vi "Create.vi"(8 "Error In":errorcluster, 11 "object in":refnum<class "WebView.lvclass">) -> (0 "Error Out":errorcluster, 3 "object out":refnum<class "WebView.lvclass">)   [LabVIEW 2024, in "WebView.lvclass"]
uses:
  <resource>/Framework/Providers/Open_GDS/ClassProviders/Provider_LvNativeClass/Templates/NativeBaseTemplate_4x4x4/NativeBaseTemplate_4x4x4.lvclass/NativeBaseTemplate_4x4x4.ctl
  WebView.lvclass
  WebView.lvclass/WebView.ctl
  <vilib>/sklein/WebView2/Webview2 Control/Paths.ctl
  <vilib>/sklein/WebView2/Webview2 Control/WebView2 Control.xctl
  <vilib>/sklein/WebView2/Webview2 Control/Core Env Options.ctl
panel:
  in  "Environment Options":T1
  in  "Path Overrides":T2
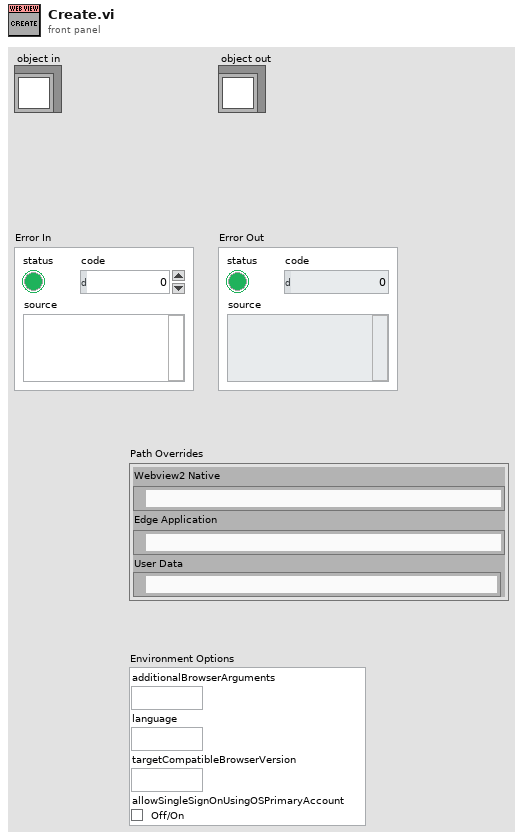
[diagram p1: front panel]
types:
  T1 = typedef "WebView2 Control.xctl/Core Env Options.ctl" = cluster{"additionalBrowserArguments":string, "language":string, "targetCompatibleBrowserVersion":string, "allowSingleSignOnUsingOSPrimaryAccount":bool}
  T2 = typedef "WebView2 Control.xctl/Paths.ctl" = cluster{"Webview2 Native":path, "Edge Application":path, "User Data":path}
  T3 = typedef "WebView.lvclass/Paths-cluster.ctl" = cluster{"Webview2 Native":path, "Edge Application":path, "User Data":path}
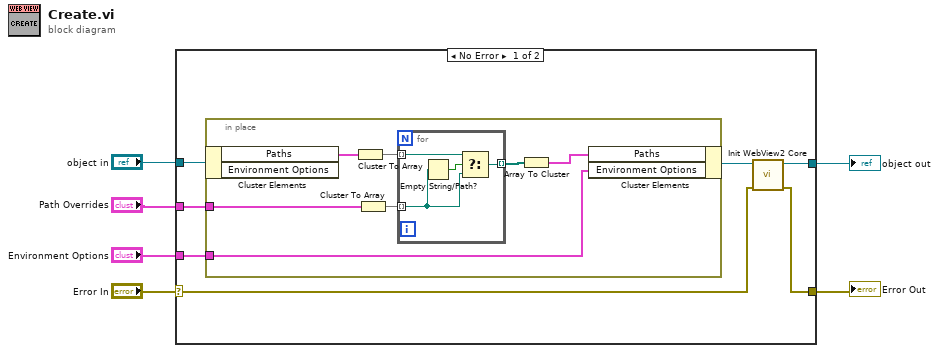
[diagram p0: block diagram]
diagram:
  n1 = case shown="No Error" "Error In" {
    selector: "Error In" -> [w9 w26]
    tunnel: [w8 w26] -> w5
    tunnel: [w12 w25] -> w3
    tunnel: "object in" -> [w13 w25]
    tunnel: "Environment Options" -> [w10 _]
    tunnel: "Path Overrides" -> [w7 _]
    frame No Error {
      n2 = in-place {
        in-place-border: w10 -> [w15]
        in-place-border: w7 -> [w14]
        n3 = in-place-cluster #1(w13) -> ("Paths"=w20:T3)  [unwired: 1 out]
        n4 = Cluster To Array(cluster=w20) -> (array=w19:path[])
        n5 = Cluster To Array(cluster=w14) -> (array=w16:path[])
        n6 = for {
          tunnel: [w24] -> w18 mode=indexing
          tunnel: w19 -> [w21] mode=indexing
          tunnel: w16 -> [w22] mode=indexing
          n7 = Empty String/Path?(string/path=w22) -> (empty?=w23:bool)
          n8 = Select(t=w21, s=w23, f=w22) -> (s? t:f=w24:path)
        }
        n9 = Array To Cluster(array=w18) -> (cluster=w17:cluster{"[0]":path, "[1]":path, "[2]":path})
        n10 = in-place-cluster #1("Paths"=w17, "Environment Options"=w15) -> (w11:refnum<class "WebView.lvclass">)
      }
      n11 = call "Init WebView2 Core.vi"("error in (no error)"=w9, "WebView 2"=w11) -> ("error out"=w8:errorcluster, "WebView out (dup)"=w12:refnum<class "WebView.lvclass">)  [unwired: 8 in]
    }
    frame Error {
    }
  }
  "Error Out" <- w5
  "object out" <- w3
